vi "Read Pressure Valve Opening (%).vi"(11 "PressureValve in":refnum<class "PressureValve.lvclass">) -> (2 "Pressure Valve Opening (%)":dbl=2.0 min=1.0 max=4.0, 3 "PressureValve out":refnum<class "PressureValve.lvclass">)   [LabVIEW 2015, in "PressureValve.lvlib" / "PressureValve.lvclass"]
uses:
  <userlib>/Common/Devices/PressureValve/PressureValve/PressureValve.lvclass
  <userlib>/Common/Devices/PressureValve/PressureValve/PressureValve.lvclass/PressureValve.ctl
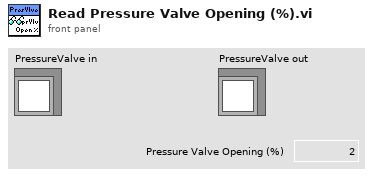
[diagram p1: front panel]
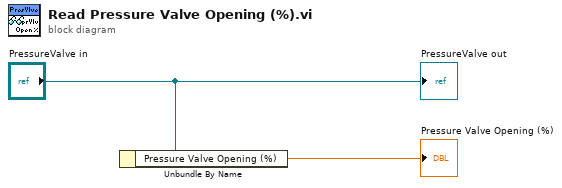
[diagram p0: block diagram]
diagram:
  n1 = Unbundle By Name("PressureValve in") -> ("Pressure Valve Opening (%)"=→"Pressure Valve Opening (%)":dbl)
  "PressureValve out" <- "PressureValve in"
